vi "Begin.vi"(8 "error in":errorcluster) -> (0 "error out":errorcluster)   [LabVIEW 2019]
doc: "Called before other user functions, this VI is expected to open initial I/O refnums, load in file data, and do all program initialization. Notice that the <B>error out</B> terminal is simply used for data flow. Wiring it to other structures or subVIs ensures that this VI runs first."
uses:
  <vilib>/Rock Robotics/SystemInterfaces/DIO/FPGA_DIOPWMChannel.ctl
  <vilib>/Rock Robotics/WPI/DriverStation/WPI_DriverStationRobotMode2.ctl
  <vilib>/Rock Robotics/WPI/Solenoid/WPI_SolenoidChannel.ctl
  <vilib>/Rock Robotics/WPI/SafetyOutput/WPI_SafetyOutputConfigMenu.ctl
  <vilib>/Rock Robotics/WPI/Joystick/WPI_JoystickDeviceEnum.ctl
  <vilib>/Rock Robotics/WPI/RobotDrive/WPI_RobotDriveOpen2MotorWithSPARK.vi
  Robot Global Data.vi
  <vilib>/Rock Robotics/Network Tables/NT Write String Array.vi
  <vilib>/Rock Robotics/WPI/RobotDrive/WPI_RobotDriveOpen2MotorWithExistingMotors.vi
  <vilib>/Rock Robotics/WPI/Utilities/WPI_GetSetVariantRefNum.vi
  <vilib>/Rock Robotics/WPI/Solenoid/WPI_SolenoidOpenSingle.vi
  <vilib>/Rock Robotics/WPI/MotorControl/WPI_MotorControlOpen SPARK.vi
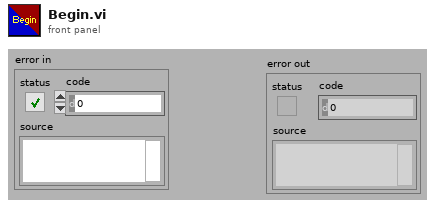
[diagram p1: front panel]
types:
  T1 = typedef "WPI_DriverStationRobotMode2.ctl" = enum16{"Autonomous Disabled", "Autonomous Enabled", "Teleop Disabled", "Teleop Enabled", "Disconnected", "Finish", "Test Disabled", "Test Enabled", "Emergency Stopped"}
  T2 = typedef "FPGA_DIOPWMChannel.ctl" = enum8{"PWM 0", "PWM 1", "PWM 2", "PWM 3", "PWM 4", "PWM 5", "PWM 6", "PWM 7", "PWM 8", "PWM 9", "PWM MXP 0", "PWM MXP 1", "PWM MXP 2", "PWM MXP 3", "PWM MXP 4", "PWM MXP 5", "PWM MXP 6", "PWM MXP 7", "PWM MXP 8", "PWM MXP 9", "Invalid"}
  T3 = typedef "WPI_SafetyOutputConfigMenu.ctl" = enum16{"Enable", "Disable"}
  T4 = typedef "WPI_MotorControlDeviceRef.ctl" = cluster{"DeviceStatus":errorcluster, "Type":T5, "PWM":cluster{"PWM Channel":T2, "DeadBand":T6}, "CAN":cluster{"Device Number":u8, "SetOutput VI Ref":variant, "GetOutput VI Ref":variant, "Enable VI Ref":variant, "Disable VI Ref":variant, "Data":variant}, "Invert":bool, "DIO PWM":cluster{"PWM \"Enable\" Channel":T2, "DIOChannel":T7, "PWM Rate":dbl}}
  T5 = typedef "WPI_MotorControlType.ctl" = enum16{"PWM", "CAN", "DIO PWM"}
  T6 = typedef "WPI_PWMDeadband.ctl" = cluster{"Name":string, "maxPositivePwm":i32, "minPositivePwm":i32, "centerPwm":i32, "maxNegativePwm":i32, "minNegativePwm":i32, "angularRange":u16}
  T7 = typedef "FPGA_DIOChannel.ctl" = enum8{"DIO 0", "DIO 1", "DIO 2", "DIO 3", "DIO 4", "DIO 5", "DIO 6", "DIO 7", "DIO 8", "DIO 9", "DIO MXP 0", "DIO MXP 1", "DIO MXP 2", "DIO MXP 3", "DIO MXP 4", "DIO MXP 5", "DIO MXP 6", "DIO MXP 7", "DIO MXP 8", "DIO MXP 9", "DIO MXP 10", "DIO MXP 11", "DIO MXP 12", "DIO MXP 13", "DIO MXP 14", "DIO MXP 15", "SPI Port CS1", "SPI Port CS2", "SPI Port CS3", "SPI Port MISO", "SPI Port MOSI", "Invalid"}
  T8 = typedef "WPI_RobotDriveDevRef.ctl" = cluster{"DevStatus":errorcluster, "Motors[]":T4[], "Square Inputs":bool, "Max Output":dbl}
  T9 = typedef "WPI_JoystickDeviceEnum.ctl" = enum16{"USB 0", "USB 1", "USB 2", "USB 3", "USB 4", "USB 5"}
  T10 = typedef "WPI_JoystickDevRef.ctl" = cluster{"Device":T9}
  T11 = typedef "WPI_SolenoidChannel.ctl" = enum8{"Solenoid 0", "Solenoid 1", "Solenoid 2", "Solenoid 3", "Solenoid 4", "Solenoid 5", "Solenoid 6", "Solenoid 7", "Invalid"}
  T12 = typedef "WPI_SolenoidDevRef.ctl" = cluster{"DevStatus":errorcluster, "Pneumatics Control Module":u8, "Forward Solenoid Channel":T11, "Reverse Solenoid Channel":T11}
  T13 = typedef "WPI_CompressorDevRef.ctl" = cluster{"DevStatus":errorcluster, "Pneumatics Control Module":u8}
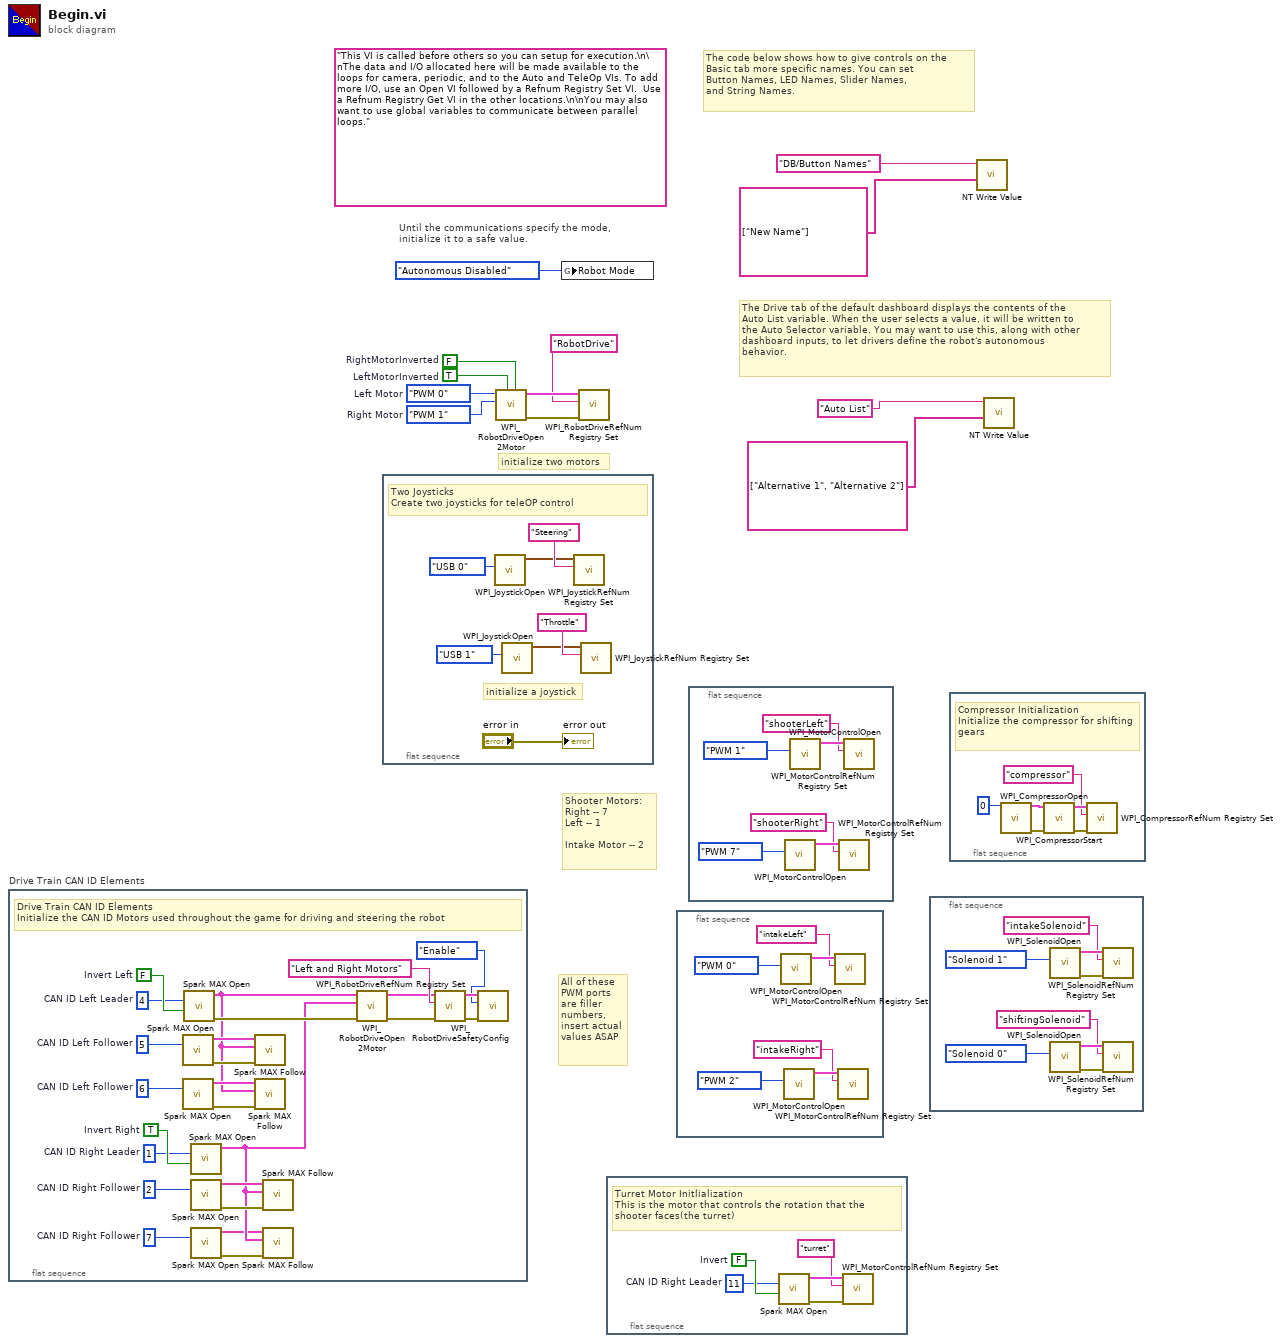
[diagram p0: block diagram]
diagram:
  (unwired) "This VI is called before others so you can setup for execution.\n\nThe data and I/O allocated here will be made available to the loops for camera, periodic, and to the Auto and TeleOp VIs. To add more I/O, use an Open VI followed by a Refnum Registry Set VI.  Use a Refnum Registry Get VI in the other locations.\n\nYou may also want to use global variables to communicate between parallel loops."
  w6 = FPGA_DIOPWMChannel."PWM 1"  # Right Motor
  w7 = FPGA_DIOPWMChannel."PWM 0"  # Left Motor
  w11 = TRUE  # LeftMotorInverted
  w12 = FALSE  # RightMotorInverted
  # "Shooter Motors:\nRight -- 7\nLeft -- 1\n\nIntake Motor -- 2"
  # "All of these\nPWM ports\nare filler \nnumbers,\ninsert actual\nvalues ASAP"
  # "The Drive tab of the default dashboard displays the contents of the\nAuto List variable. When the user selects a value, it will be written to\nthe Auto Selector variable. You may want to use this, along with other\ndashboard inputs, to let drivers define the robot's autonomous\nbehavior."
  # "The code below shows how to give controls on the\nBasic tab more specific names. You can set\nButton Names, LED Names, Slider Names,\nand String Names."
  # "Until the communications specify the mode,\ninitialize it to a safe value."
  # "initialize two motors"
  n1 = flat-sequence "Drive Train CAN ID Elements" {
    frame #0 {
      w16 = u8 7  # CAN ID Right Follower
      w21 = u8 6  # CAN ID Left Follower
      w37 = FALSE  # Invert Left
      w36 = TRUE  # Invert Right
      w29 = u8 1  # CAN ID Right Leader
      w30 = u8 2  # CAN ID Right Follower
      w23 = u8 4  # CAN ID Left Leader
      w22 = u8 5  # CAN ID Left Follower
      # "Drive Train CAN ID Elements\nInitialize the CAN ID Motors used throughout the game for driving and steering the robot"
      n2 = call <vilib>:"Spark MAX Open.vi"("Device Number"=w22) -> ("error out"=w26:errorcluster, "MotorControlDeviceRef"=w25:T4)  [unwired: 9 in]
      n3 = call <vilib>:"Spark MAX Open.vi"("Device Number"=w21) -> ("error out"=w19:errorcluster, "MotorControlDeviceRef"=w20:T4)  [unwired: 9 in]
      n4 = call <vilib>:"Spark MAX Open.vi"("Invert"=w37, "Device Number"=w23) -> ("error out"=w24:errorcluster, "MotorControlDeviceRef"=w18:T4)  [unwired: 8 in]
      n5 = call <vilib>:"Spark MAX Open.vi"("Invert"=w36, "Device Number"=w29) -> ("MotorControlDeviceRef"=w15:T4)  [unwired: 8 in, 1 out]
      n6 = call <vilib>:"Spark MAX Open.vi"("Device Number"=w30) -> ("error out"=w27:errorcluster, "MotorControlDeviceRef"=w28:T4)  [unwired: 9 in]
      n7 = call <vilib>:"Spark MAX Open.vi"("Device Number"=w16) -> ("error out"=w17:errorcluster, "MotorControlDeviceRef"=w14:T4)  [unwired: 9 in]
      n8 = call <vilib>:"Spark MAX Follow.vi"("error in (no error)"=w26, "Master Controller"=w18, "MotorControlDeviceRef"=w25) -> ()  [unwired: 7 in, 2 out]
      n9 = call <vilib>:"Spark MAX Follow.vi"("error in (no error)"=w19, "Master Controller"=w18, "MotorControlDeviceRef"=w20) -> ()  [unwired: 7 in, 2 out]
      n10 = call <vilib>:"Spark MAX Follow.vi"("error in (no error)"=w27, "Master Controller"=w15, "MotorControlDeviceRef"=w28) -> ()  [unwired: 7 in, 2 out]
      n11 = call <vilib>:"Spark MAX Follow.vi"("error in (no error)"=w17, "Master Controller"=w15, "MotorControlDeviceRef"=w14) -> ()  [unwired: 7 in, 2 out]
      n12 = call-poly <vilib>:"WPI_RobotDriveOpen2Motor.vi"("error in (no error)"=w24, "Right Motor Dev Ref"=w15, "Left Motor Dev Ref"=w18) -> ("error out"=w33:errorcluster, "RobotDriveDevRef"=w31:T8)  [unwired: 7 in]
      n13 = call <vilib>:"WPI_RobotDriveRefNum Registry Set.vi"("error in (no error)"=w33, "refnum name"="Left and Right Motors", "RobotDriveDevRef"=w31) -> ("error out"=w35:errorcluster, "RobotDriveDevRef"=w34:T8)  [unwired: 7 in]
      n14 = call <vilib>:"WPI_RobotDriveSafetyConfig.vi"("error in (no error)"=w35, "mode"=WPI_SafetyOutputConfigMenu."Enable", "RobotDriveDevRef"=w34) -> ()  [unwired: 7 in, 2 out]
    }
  }
  n15 = flat-sequence {
    frame #0 {
      # "initialize a joystick"
      # "Two Joysticks\nCreate two joysticks for teleOP control"
      n16 = call <vilib>:"WPI_JoystickOpen.vi"("JoystickDevice"=WPI_JoystickDeviceEnum."USB 0") -> ("JoystickDevRef"=w43:T10)  [unwired: 10 in]
      n17 = call <vilib>:"WPI_JoystickOpen.vi"("JoystickDevice"=WPI_JoystickDeviceEnum."USB 1") -> ("JoystickDevRef"=w40:T10)  [unwired: 10 in]
      n18 = call <vilib>:"WPI_JoystickRefNum Registry Set.vi"("refnum name"="Steering", "JoystickDevRef"=w43) -> ()  [unwired: 8 in, 2 out]
      n19 = call <vilib>:"WPI_JoystickRefNum Registry Set.vi"("refnum name"="Throttle", "JoystickDevRef"=w40) -> ()  [unwired: 8 in, 2 out]
      "error out" <- "error in"
    }
  }
  n20 = call-poly <vilib>:"WPI_RobotDriveOpen2Motor.vi"("Right Motor Inverted"=w12, "Left Motor Inverted"=w11, "Right Motor"=w6, "Left Motor"=w7) -> ("error out"=w8:errorcluster, "RobotDriveDevRef"=w10:T8)  [unwired: 1 in, 5 out]
  n21 = global write "Robot Global Data.vi" "Robot Mode"(WPI_DriverStationRobotMode2."Autonomous Disabled" ("Robot Mode")) -> ()
  n22 = call <vilib>:"WPI_RobotDriveRefNum Registry Set.vi"("error in (no error)"=w8, "refnum name"="RobotDrive", "RobotDriveDevRef"=w10) -> ()  [unwired: 1 in, 8 out]
  n23 = flat-sequence {
    frame #0 {
      w49 = FALSE  # Invert
      w48 = u8 11  # CAN ID Right Leader
      # "Turret Motor Initlialization\nThis is the motor that controls the rotation that the shooter faces(the turret)"
      n24 = call <vilib>:"Spark MAX Open.vi"("Invert"=w49, "Device Number"=w48) -> ("error out"=w46:errorcluster, "MotorControlDeviceRef"=w47:T4)  [unwired: 8 in]
      n25 = call <vilib>:"WPI_MotorControlRefNum Registry Set.vi"("error in (no error)"=w46, "refnum name"="turret", "MotorControlDevRef"=w47) -> ()  [unwired: 7 in, 2 out]
    }
  }
  n26 = flat-sequence {
    frame #0 {
      n27 = call-poly <vilib>:"WPI_MotorControlOpen.vi"("PWM Channel"=FPGA_DIOPWMChannel."PWM 0") -> ("MotorControlDeviceRef"=w54:T4)  [unwired: 9 in, 1 out]
      n28 = call-poly <vilib>:"WPI_MotorControlOpen.vi"("PWM Channel"=FPGA_DIOPWMChannel."PWM 2") -> ("MotorControlDeviceRef"=w51:T4)  [unwired: 9 in, 1 out]
      n29 = call <vilib>:"WPI_MotorControlRefNum Registry Set.vi"("refnum name"="intakeLeft", "MotorControlDevRef"=w54) -> ()  [unwired: 8 in, 2 out]
      n30 = call <vilib>:"WPI_MotorControlRefNum Registry Set.vi"("refnum name"="intakeRight", "MotorControlDevRef"=w51) -> ()  [unwired: 8 in, 2 out]
    }
  }
  n31 = flat-sequence {
    frame #0 {
      n32 = call-poly <vilib>:"WPI_MotorControlOpen.vi"("PWM Channel"=FPGA_DIOPWMChannel."PWM 7") -> ("MotorControlDeviceRef"=w57:T4)  [unwired: 9 in, 1 out]
      n33 = call-poly <vilib>:"WPI_MotorControlOpen.vi"("PWM Channel"=FPGA_DIOPWMChannel."PWM 1") -> ("MotorControlDeviceRef"=w60:T4)  [unwired: 9 in, 1 out]
      n34 = call <vilib>:"WPI_MotorControlRefNum Registry Set.vi"("refnum name"="shooterRight", "MotorControlDevRef"=w57) -> ()  [unwired: 8 in, 2 out]
      n35 = call <vilib>:"WPI_MotorControlRefNum Registry Set.vi"("refnum name"="shooterLeft", "MotorControlDevRef"=w60) -> ()  [unwired: 8 in, 2 out]
    }
  }
  n36 = flat-sequence {
    frame #0 {
      n37 = call-poly <vilib>:"WPI_SolenoidOpen.vi"("Solenoid Channel"=WPI_SolenoidChannel."Solenoid 1") -> ("error out"=w68:errorcluster, "SolenoidDevRef"=w69:T12)  [unwired: 2 in, 7 out]
      n38 = call-poly <vilib>:"WPI_SolenoidOpen.vi"("Solenoid Channel"=WPI_SolenoidChannel."Solenoid 0") -> ("error out"=w64:errorcluster, "SolenoidDevRef"=w65:T12)  [unwired: 2 in, 7 out]
      n39 = call <vilib>:"WPI_SolenoidRefNum Registry Set.vi"("error in (no error)"=w68, "refnum name"="intakeSolenoid", "SolenoidDevRef"=w69) -> ()  [unwired: 7 in, 2 out]
      n40 = call <vilib>:"WPI_SolenoidRefNum Registry Set.vi"("error in (no error)"=w64, "refnum name"="shiftingSolenoid", "SolenoidDevRef"=w65) -> ()  [unwired: 7 in, 2 out]
    }
  }
  n41 = flat-sequence {
    frame #0 {
      # "Compressor Initialization\nInitialize the compressor for shifting gears"
      n42 = call <vilib>:"WPI_CompressorOpen.vi"("Pneumatics Control Module (0)"=u8 0) -> ("CompressorDevRef"=w75:T13, "error out"=w74:errorcluster)  [unwired: 13 in]
      n43 = call <vilib>:"WPI_CompressorStart.vi"("error in (no error)"=w74, "CompressorDevRef"=w75) -> ("error out"=w72:errorcluster, "CompressorDevRef"=w71:T13)  [unwired: 8 out]
      n44 = call <vilib>:"WPI_CompressorRefNum Registry Set.vi"("error in (no error)"=w72, "refnum name"="compressor", "CompressorDevRef"=w71) -> ()  [unwired: 7 in, 2 out]
    }
  }
  n45 = call-poly <vilib>:"NT Write Value.vi"("String Array"=string[] ["New Name"], "Name"="DB/Button Names") -> ()  [unwired: 9 in, 1 out]
  n46 = call-poly <vilib>:"NT Write Value.vi"("String Array"=string[] ["Alternative 1", "Alternative 2"], "Name"="Auto List") -> ()  [unwired: 9 in, 1 out]
